vi "ShuttleValveON_OFF.vi"(9 "gradient enabled":bool=TRUE, 10 "elapsed time (ms)":u32, 11 "gradient parameters":T1) -> (2 "x < y?":bool)   [LabVIEW 2014]
uses:
  <vilib>/ptbypt/NI_PtbyPt.lvlib
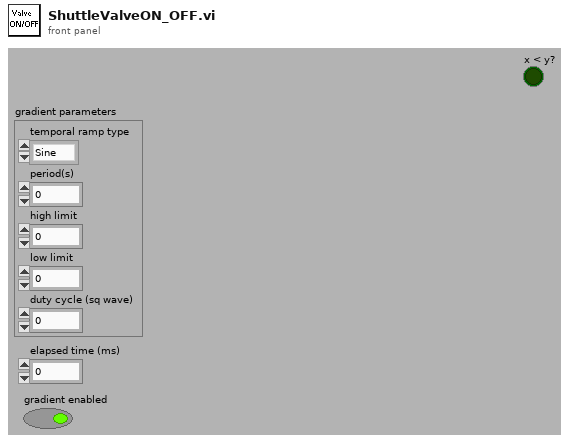
[diagram p1: front panel]
types:
  T1 = cluster{"temporal ramp type":enum16{"Sine", "Triangle", "Sawtooth", "Square", "Exponential"}, "period(s)":dbl, "high limit":dbl, "low limit":dbl, "duty cycle (sq wave)":dbl}
  T2 = enum16{"Sine", "Triangle", "Sawtooth", "Square", "Exponential"}
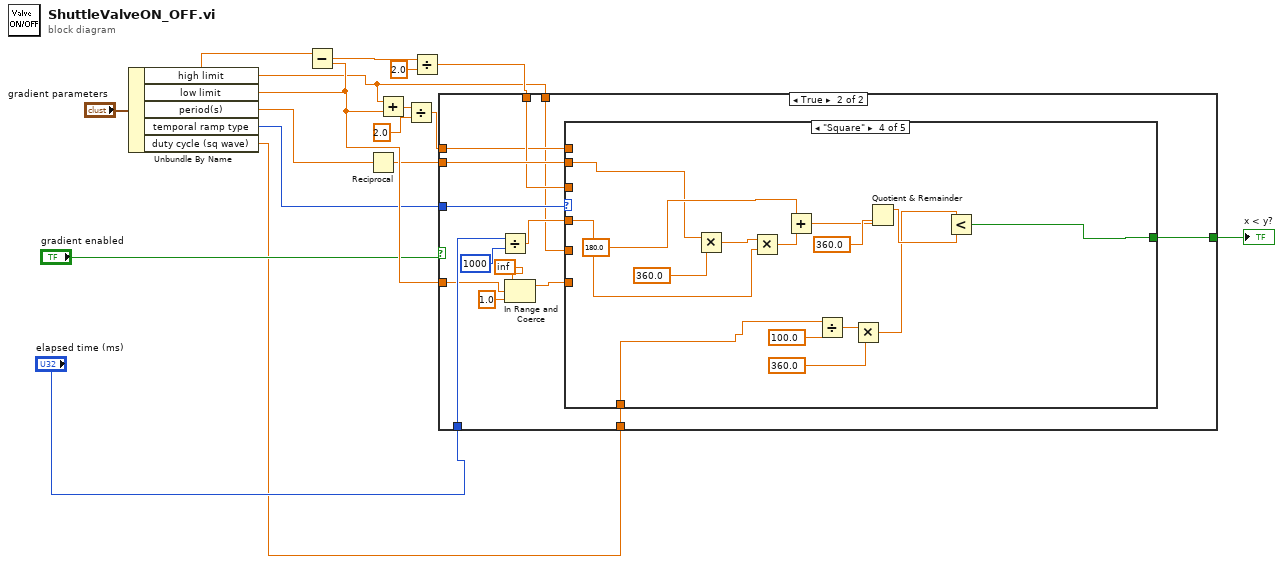
[diagram p0: block diagram]
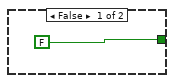
[diagram p2: hidden frame]
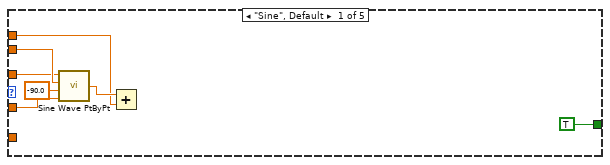
[diagram p3: hidden frame]
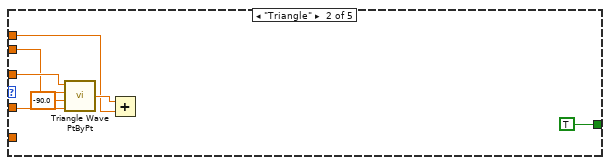
[diagram p4: hidden frame]
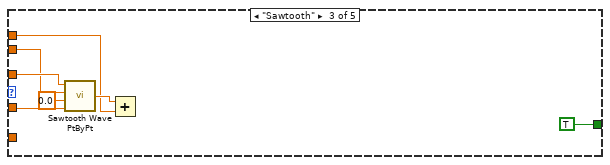
[diagram p5: hidden frame]
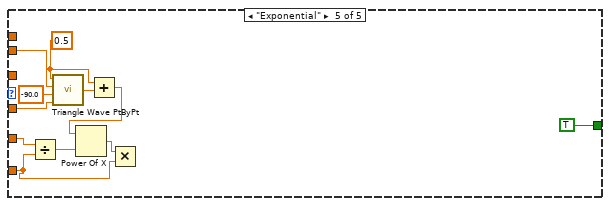
[diagram p6: hidden frame]
diagram:
  n1 = Unbundle By Name("gradient parameters") -> ("high limit"=w13:dbl, "low limit"=w16:dbl, "period(s)"=w11:dbl, "temporal ramp type"=w15:T2, "duty cycle (sq wave)"=w2:dbl)
  n2 = Subtract(x=w13, y=w16) -> (x-y=w7:dbl)
  n3 = Reciprocal(x=w11) -> (1/x=w6:dbl)
  n4 = Add(x=w13, y=w16) -> (x+y=w8:dbl)
  n5 = Divide(x=w8, y=2.0) -> (x/y=w10:dbl)
  n6 = Divide(x=w7, y=2.0) -> (x/y=w14:dbl)
  n7 = case shown="True" "gradient enabled" {
    tunnel: "elapsed time (ms)" -> [_ w31]
    tunnel: w6 -> [_ w28]
    tunnel: w14 -> [_ w27]
    tunnel: w10 -> [_ w26]
    tunnel: w15 -> [_ w25]
    tunnel: w16 -> [_ w22]
    tunnel: w13 -> [_ w24]
    tunnel: w2 -> [_ w20]
    tunnel: [FALSE w18] -> w1
    frame False {
    }
    frame True {
      n8 = Divide(x=w31, y=u32 1000) -> (x/y=w30:dbl)
      n9 = In Range and Coerce(upper limit=inf, x=w22, lower limit=1.0) -> (coerced(x)=w23:dbl)  [unwired: 1 out]
      n10 = case shown="\"Square\"" w25 {
        tunnel: w30 -> [w38 w41 w48 w57 w78]
        tunnel: w28 -> [w37 w43 w50 w55 w76]
        tunnel: w27 -> [w35 w44 w51 _ _]
        tunnel: w26 -> [w33 w42 w49 _ _]
        tunnel: w23 -> [_ _ _ _ w69]
        tunnel: w24 -> [_ _ _ _ w73]
        tunnel: w20 -> [_ _ _ w54 _]
        tunnel: [TRUE TRUE TRUE w53 TRUE] -> w18
        frame "Sine", Default {
          n11 = call <vilib>:"Sine Wave PtByPt.vi"("time"=w38, "phase"=-90.0, "frequency"=w37, "amplitude"=w35) -> ("sine wave"=w34:dbl)
          n12 = Add(x=w34, y=w33) -> ()  [unwired: 1 out]
        }
        frame "Triangle" {
          n13 = call <vilib>:"Triangle Wave PtByPt.vi"("time"=w41, "phase"=-90.0, "frequency"=w43, "amplitude"=w44) -> ("triangle wave"=w45:dbl)
          n14 = Add(x=w45, y=w42) -> ()  [unwired: 1 out]
        }
        frame "Sawtooth" {
          n15 = call <vilib>:"Sawtooth Wave PtByPt.vi"("time"=w48, "phase"=0.0, "frequency"=w50, "amplitude"=w51) -> ("sawtooth wave"=w52:dbl)
          n16 = Add(x=w52, y=w49) -> ()  [unwired: 1 out]
        }
        frame "Square" {
          n17 = Multiply(x=w55, y=360.0 ("x")) -> (x*y=w58:dbl)
          n18 = Multiply(x=w58, y=w57) -> (x*y=w60:dbl)
          n19 = Add(x=180.0 ("phase"), y=w60) -> (x+y=w61:dbl)
          n20 = Divide(x=w54, y=100.0) -> (x/y=w63:dbl)
          n21 = Multiply(x=w63, y=360.0) -> (x*y=w64:dbl)
          n22 = Quotient & Remainder(x=w61, y=360.0) -> (x-y*floor(x/y)=w65:dbl)  [unwired: 1 out]
          n23 = Less?(x=w65, y=w64) -> (x < y?=w53:bool)
        }
        frame "Exponential" {
          w74 = 0.5 ("amplitude")
          n24 = Divide(x=w73, y=w69) -> (x/y=w72:dbl)
          n25 = call <vilib>:"Triangle Wave PtByPt.vi"("time"=w78, "phase"=-90.0, "frequency"=w76, "amplitude"=w74) -> ("triangle wave"=w75:dbl)
          n26 = Add(x=w74, y=w75) -> (x+y=w71:dbl)
          n27 = Power Of X(1:w72, 2:w71) -> (0:w70:dbl)
          n28 = Multiply(x=w70, y=w69) -> ()  [unwired: 1 out]
        }
      }
    }
  }
  "x < y?" <- w1
